vi "daqio_Compact_Write_Multiple_single_Timestamp.vi"(6 "Use Server Time (UTC)?":bool, 7 "daq.io Device Channel Indexes":u32[](array[numeric]), 8 "error in (no error)":errorcluster, 9 "Timestamp":timestamp, 10 "Values":dbl[](array[numeric]), 11 "daq.io type in":T1={"daq.io ref"=refnum, "daq.io API Base"="http://dashboard.daq.io/api/v1", "Device Key"="", "Account ID"="", "online"=TRUE, "SSL"=FALSE, "buffer"=TRUE}) -> (0 "error out":errorcluster, 3 "daq.io type out":T1={"daq.io ref"=refnum, "daq.io API Base"="http://dashboard.daq.io/api/v1", "Device Key"="", "Account ID"="", "online"=TRUE, "SSL"=FALSE, "buffer"=TRUE})   [LabVIEW 2013, in "daqio minimal.lvlib"]
doc: "This VI writes multiple data points to a channel of a daq.io device with the same time stamp. \n\nIf the daq.io Device Channel does not exist online, a new channel will be auto-created and data will be stored there. You have to provide a Channel Key where the value will be written to."
uses:
  daqio minimal.lvlib
  _typedefs/daqio-Type.ctl
  <vilib>/httpClient/ClientHandle.ctl
  _typedefs/daqio-Buffer-Commands.ctl
  _typedefs/connection_FGV_commands.ctl
  <vilib>/Easy HTTP Client/Easy HTTP.lvlib
  <vilib>/httpClient/LabVIEWHTTPClient.lvlib
panel:
  out "JSON string":string
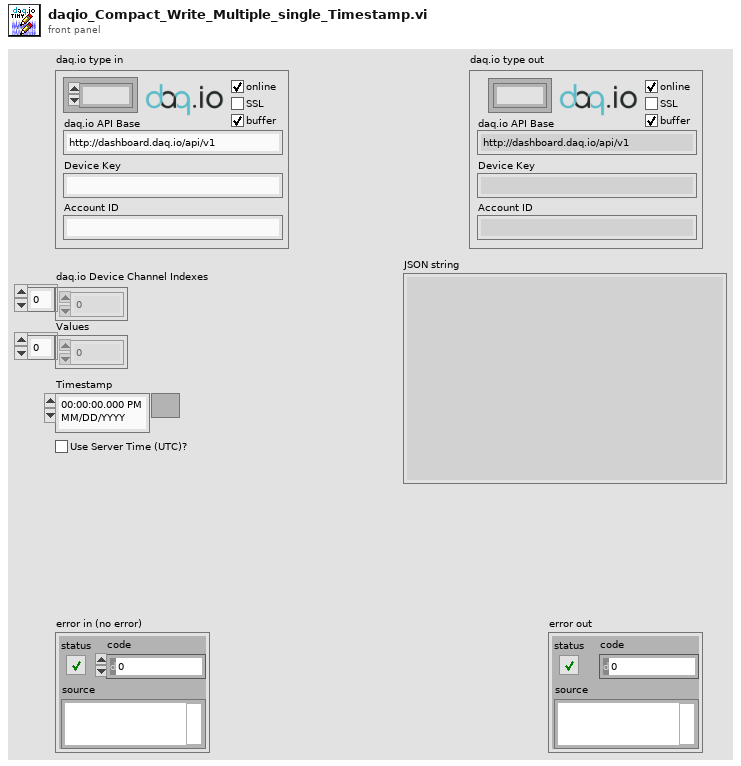
[diagram p1: front panel]
types:
  T1 = typedef "daqio minimal.lvlib/daqio-Type.ctl" = cluster{"daq.io ref":T2, "daq.io API Base":string, "Device Key":string, "Account ID":string, "online":bool, "SSL":bool, "buffer":bool}
  T2 = typedef "LabVIEWHTTPClient.lvlib/ClientHandle.ctl" = refnum<k1>
  T3 = typedef "daqio minimal.lvlib/daqio-Buffer-Commands.ctl" = enum16{"Add to Buffer", "Post from Buffer", "Clear Buffer", "Init"}
  T4 = typedef "daqio minimal.lvlib/connection_FGV_commands.ctl" = enum16{"Set Conn Stat", "Save Key", "Get Key from File", "Set Type", "Set Buffer", "Get"}
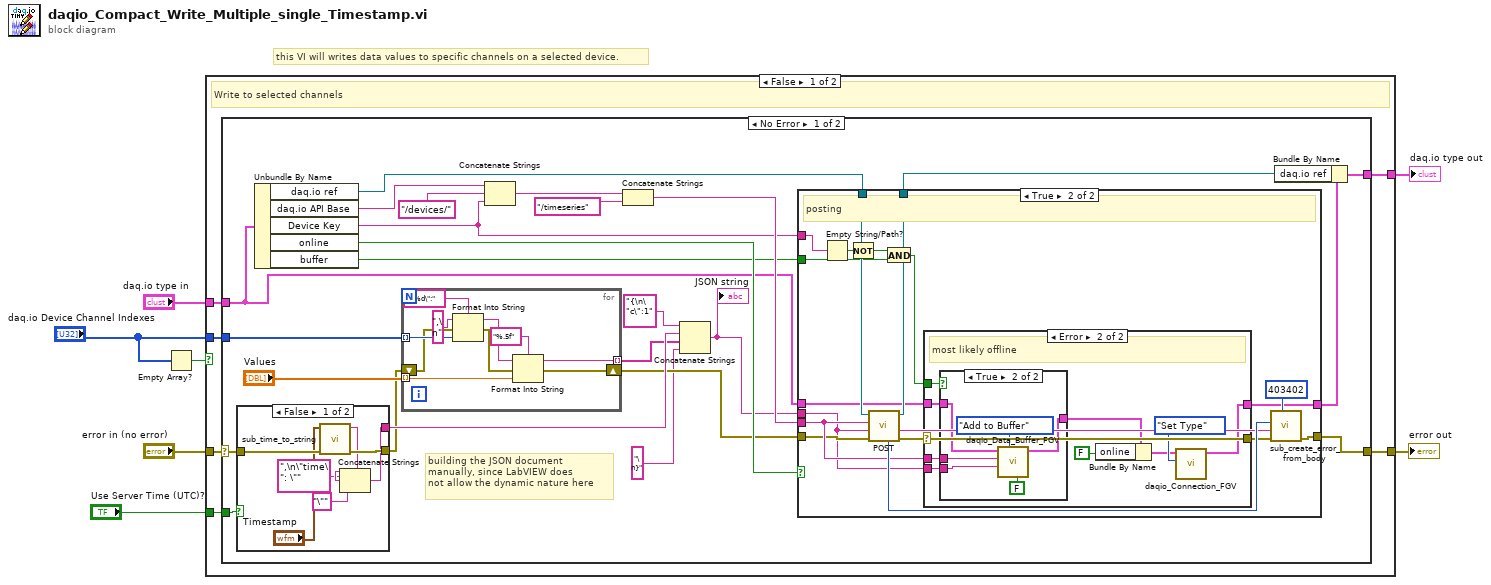
[diagram p0: block diagram]
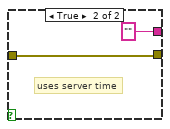
[diagram p2: hidden frame]
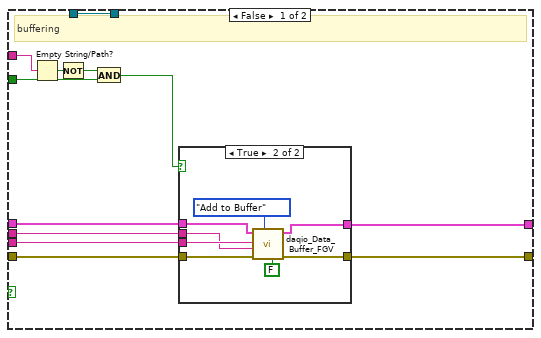
[diagram p3: hidden frame]
diagram:
  # "this VI will writes data values to specific channels on a selected device."
  n1 = Empty Array?(array="daq.io Device Channel Indexes") -> (empty?=w4:bool)
  n2 = case shown="False" w4 {
    tunnel: "daq.io type in" -> [w13 w120]
    tunnel: [w12 w120] -> w7
    tunnel: [w11 w119] -> w6
    tunnel: "error in (no error)" -> [w10 w119]
    tunnel: "daq.io Device Channel Indexes" -> [w9 _]
    tunnel: "Use Server Time (UTC)?" -> [w8 _]
    frame False {
      # "Write to selected channels"
      n3 = case shown="No Error" w10 {
        selector: w10 -> [w31 w117]
        tunnel: w13 -> [w26 w118]
        tunnel: [w29 w118] -> w12
        tunnel: [w32 w117] -> w11
        tunnel: w9 -> [w23 _]
        tunnel: w8 -> [w21 _]
        frame No Error {
          # "building the JSON document \nmanually, since LabVIEW does\nnot allow the dynamic nature here"
          n4 = case shown="False" w21 {
            tunnel: w31 -> [w45 w46]
            tunnel: [w41 "" ("time")] -> w19
            tunnel: [w43 w46] -> w17
            frame False {
              n5 = call "sub_time_to_string.vi"("error in (no error)"=w45, "timestamp"="Timestamp") -> ("error out"=w43:errorcluster, "time"=w42:string)  [unwired: 8 in]
              n6 = Concatenate Strings(",\n\"time\": \"" ("string"), w42, "\"" ("string")) -> (w41:string)
            }
            frame True {
              # "uses server time"
            }
          }
          n7 = Unbundle By Name(w26) -> ("daq.io ref"=w33:T2, "daq.io API Base"=w38:string, "Device Key"=w24:string, "online"=w30:bool, "buffer"=w25:bool)
          n8 = for {
            tunnel: "Values" -> [w55] mode=indexing
            tunnel: w23 -> [w57] mode=indexing
            tunnel: [w52] -> w15 mode=indexing
            shift-right: [w49] -> w18
            shift-left: w17 -> [w48]
            n9 = Format Into String(format string="\"%d\":", initial string=",\n", error in=w48, w57) -> (resulting string=w54:string, error out=w50:errorcluster)
            n10 = Format Into String(format string="%.5f", initial string=w54, error in=w50, w55) -> (resulting string=w52:string, error out=w49:errorcluster)
          }
          n11 = Concatenate Strings(w38, "/devices/", w24) -> (w34:string)
          n12 = Concatenate Strings(w34, "/timeseries") -> (w35:string)
          n13 = Concatenate Strings("{\n\"c\":1" ("string"), w19, w15, "\n}") -> (w14:string)
          "JSON string" <- w14
          n14 = case shown="True" w30 {
            tunnel: [w69 w97] -> w37
            tunnel: w35 -> [w67 w89]
            tunnel: w33 -> [w69 w96]
            tunnel: [w68 w95] -> w32
            tunnel: w26 -> [w66 w90]
            tunnel: [w65 w87] -> w28
            tunnel: w25 -> [w61 w83]
            tunnel: w24 -> [w62 w84]
            tunnel: w18 -> [w58 w81]
            tunnel: w14 -> [w59 w80]
            frame False {
              # "buffering"
              n15 = Empty String/Path?(string/path=w62) -> (empty?=w64:bool)
              n16 = Not(x=w64) -> (.not. x?=w63:bool)
              n17 = And(x=w63, y=w61) -> (x .and. y?=w60:bool)
              n18 = case shown="True" w60 {
                tunnel: [w70 w79] -> w68
                tunnel: w67 -> [_ w78]
                tunnel: w66 -> [w71 w76]
                tunnel: [w71 w74] -> w65
                tunnel: w58 -> [w70 w73]
                tunnel: w59 -> [_ w72]
                frame False {
                }
                frame True {
                  n19 = call "daqio_Data_Buffer_FGV.vi"("Is Array?"=FALSE, "Buffer Command"=daqio-Buffer-Commands."Add to Buffer", "error in (no error)"=w73, "JSON Data"=w72, "API route"=w78, "daq.io type in"=w76) -> ("error out"=w79:errorcluster, "daq.io type out"=w74:T1)  [unwired: 4 in]
                }
              }
            }
            frame True {
              # "posting"
              n20 = Empty String/Path?(string/path=w84) -> (empty?=w85:bool)
              n21 = Not(x=w85) -> (.not. x?=w86:bool)
              n22 = call <vilib>:"POST.vi"("error in (no error)"=w81, "data"=w80, "url"=w89, "client handle"=w96) -> ("error out"=w91:errorcluster, "body"=w92:string, "client handle out"=w97:T2, "HTTP Response Code"=w94:i32)  [unwired: 3 in, 1 out]
              n23 = And(x=w86, y=w83) -> (x .and. y?=w82:bool)
              n24 = case shown="Error" w91 {
                selector: w91 -> [w99 w109]
                tunnel: [w99 w109] -> w88
                tunnel: w90 -> [w98 w103]
                tunnel: w89 -> [_ w104]
                tunnel: [w98 w102] -> w87
                tunnel: w82 -> [_ w101]
                tunnel: w80 -> [_ w100]
                frame No Error {
                }
                frame Error {
                  # "most likely offline"
                  n25 = case shown="True" w101 {
                    tunnel: [w110 w115] -> w107
                    tunnel: w104 -> [_ w114]
                    tunnel: w103 -> [w110 w112]
                    tunnel: w100 -> [_ w111]
                    frame False {
                    }
                    frame True {
                      n26 = call "daqio_Data_Buffer_FGV.vi"("Is Array?"=FALSE, "Buffer Command"=daqio-Buffer-Commands."Add to Buffer", "JSON Data"=w111, "API route"=w114, "daq.io type in"=w112) -> ("daq.io type out"=w115:T1)  [unwired: 5 in, 1 out]
                    }
                  }
                  n27 = Bundle By Name(cluster=w107, "online"=FALSE) -> (w105:T1)
                  n28 = call "daqio_Connection_FGV.vi"("Command"=connection_FGV_commands."Set Type" ("Enum"), "daq.io type in"=w105) -> ("daq.io type out"=w102:T1)  [unwired: 6 in, 3 out]
                }
              }
              n29 = call "sub_create_error_from_body.vi"("error code"=403402, "error in (no error)"=w88, "http code"=w94, "body"=w92) -> ("error out"=w95:errorcluster)  [unwired: 7 in]
            }
          }
          n30 = Bundle By Name(cluster=w28, "daq.io ref"=w37) -> (w29:T1)
        }
        frame Error {
        }
      }
    }
    frame True {
      # "no Channel Key: nothing to do"
    }
  }
  "error out" <- w6
  "daq.io type out" <- w7
